vi "Get Shared Data Dir.vi"() -> (0 "Error Out":errorcluster, 3 "Data Directory Path":path)   [LabVIEW 2019]
doc: "Returns path to a shared data directory on all platforms. Creates intermediate directories if necessary with read/write access\nScott Hannahs <sth@magnet.fsu.edu>"
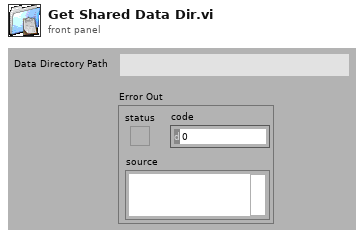
[diagram p1: front panel]
types:
  T1 = enum16{"CSIDL_DESKTOP", "CSIDL_INTERNET", "CSIDL_PROGRAMS", "CSIDL_CONTROLS", "CSIDL_PRINTERS\n", "CSIDL_PERSONAL", "CSIDL_FAVORITES", "CSIDL_STARTUP", "CSIDL_RECENT", "CSIDL_SENDTO", "CSIDL_BITBUCKET", "CSIDL_STARTMENU", "DUMMY1", "DUMMY2", "DUMMY3", "DUMMY4", "CSIDL_DESKTOPDIRECTORY", "CSIDL_DRIVES", "CSIDL_NETWORK", "CSIDL_NETHOOD", "CSIDL_FONTS", "CSIDL_TEMPLATES", "CSIDL_COMMON_STARTMENU", "CSIDL_COMMON_PROGRAMS", "CSIDL_COMMON_STARTUP", "CSIDL_COMMON_DESKTOPDIRECTORY", "CSIDL_APPDATA", "CSIDL_PRINTHOOD", "CSIDL_LOCAL_APPDATA", "CSIDL_ALTSTARTUP", "CSIDL_COMMON_ALTSTARTUP", "CSIDL_COMMON_FAVORITES", "CSIDL_INTERNET_CACHE", "CSIDL_COOKIES", "CSIDL_HISTORY", "CSIDL_COMMON_APPDATA", "CSIDL_WINDOWS", "CSIDL_SYSTEM", "CSIDL_PROGRAM_FILES", "CSIDL_MYPICTURES", "CSIDL_PROFILE", "CSIDL_SYSTEMX86", "CSIDL_PROGRAM_FILESX86", "CSIDL_PROGRAM_FILES_COMMON", "CSIDL_PROGRAM_FILES_COMMONX86", "CSIDL_COMMON_TEMPLATES", "CSIDL_COMMON_DOCUMENTS", "CSIDL_COMMON_ADMINTOOLS", "CSIDL_ADMINTOOLS"}
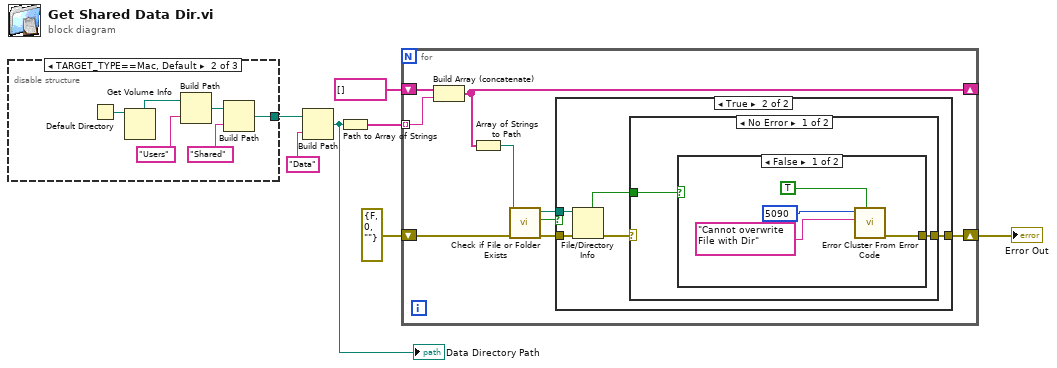
[diagram p0: block diagram]
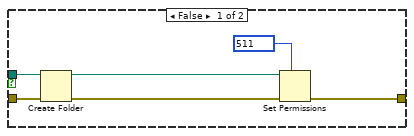
[diagram p2: hidden frame]
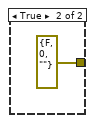
[diagram p3: hidden frame]
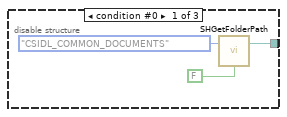
[diagram p5: hidden frame]
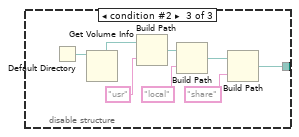
[diagram p6: hidden frame]
diagram:
  n1 = disable-structure shown="TARGET_TYPE==Mac, Default" {
    disable-tunnel: [w8 w11 w19] -> w4
    frame condition #0 {
      n2 = call "SHGetFolderPath.vi"("Return Current Path:F / Default Path:T (F)"=FALSE, "CSIDL"=T1."CSIDL_COMMON_DOCUMENTS") -> ("Path"=w8:path)  [unwired: 2 in, 1 out]
    }
    frame condition #1 (active) {
      n3 = Default Directory() -> (w13:path)
      n4 = Get Volume Info(11:w13) -> (5:w12:path)  [unwired: 1 in, 5 out]
      n5 = Build Path(base path=w12, name or relative path="Users") -> (appended path=w14:path)
      n6 = Build Path(base path=w14, name or relative path="Shared") -> (appended path=w11:path)
    }
    frame condition #2 {
      n7 = Default Directory() -> (w17:path)
      n8 = Get Volume Info(11:w17) -> (5:w21:path)  [unwired: 1 in, 5 out]
      n9 = Build Path(base path=w21, name or relative path="usr") -> (appended path=w22:path)
      n10 = Build Path(base path=w22, name or relative path="local") -> (appended path=w20:path)
      n11 = Build Path(base path=w20, name or relative path="share") -> (appended path=w19:path)
    }
  }
  n12 = Build Path(base path=w4, name or relative path="Data") -> (appended path=w2:path)
  "Data Directory Path" <- w2
  n13 = Path to Array of Strings(0:w2) -> (2:w7:string[])  [unwired: 1 out]
  n14 = for {
    tunnel: w7 -> [w33] mode=indexing
    shift-right: [w31] -> _
    shift-left: string[] [] -> [w32]
    shift-right: [w25] -> w3
    shift-left: errorcluster {"status"=FALSE, "code"=0, "source"=""} ("error IO") -> [w26]
    n15 = Build Array (concatenate)(w32, w33) -> (w31:string[])
    n16 = Array of Strings to Path(0:w31) -> (2:w30:path)  [unwired: 1 in]
    n17 = call <vilib>:"Check if File or Folder Exists.vi"("error in (no error)"=w26, "path"=w30) -> ("error out"=w27:errorcluster, "file or folder exists?"=w29:bool, "dup path"=w28:path)  [unwired: 7 in]
    n18 = case shown="True" w29 {
      tunnel: w28 -> [w39 w43]
      tunnel: w27 -> [w38 w44]
      tunnel: [w34 w41] -> w25
      frame False {
        n19 = Create Folder(path (use dialog)=w39, error in=w38) -> (created path=w37:path, error out=w36:errorcluster)  [unwired: 1 in, 1 out]
        n20 = Set Permissions(7:i16 511 ("permissions"), 8:w36, 11:w37) -> (0:w34:errorcluster)  [unwired: 2 in, 1 out]
      }
      frame True {
        n21 = File/Directory Info(path=w43, error in=w44) -> (directory=w40:bool, error out=w42:errorcluster)  [unwired: 5 out]
        n22 = case shown="No Error" w42 {
          selector: w42 -> [_ w52]
          tunnel: [w46 w52] -> w41
          tunnel: w40 -> [w45 _]
          frame No Error {
            n23 = case shown="False" w45 {
              tunnel: [w47 errorcluster {"status"=FALSE, "code"=0, "source"=""} ("error out")] -> w46
              frame False {
                n24 = call <vilib>:"Error Cluster From Error Code.vi"("show call chain? (False)"=TRUE, "error message (\"\")"="Cannot overwrite File with Dir" ("error message (\"\")"), "error code (0)"=5090 ("code")) -> ("error out"=w47:errorcluster)  [unwired: 6 in]
              }
              frame True {
              }
            }
          }
          frame Error {
          }
        }
      }
    }
  }
  "Error Out" <- w3
